vi "I-O Test.vi"() -> ()   [LabVIEW 2019]
uses:
  Classes/Controller/I-O/I-O.lvclass
  Classes/Controller/Controller.lvclass
panel:
  out "channel":dbl
  in  "Type":i32
  in  "Position":i32
  in  "Region":i32
  in  "Value":bool
  in  "Stop":bool
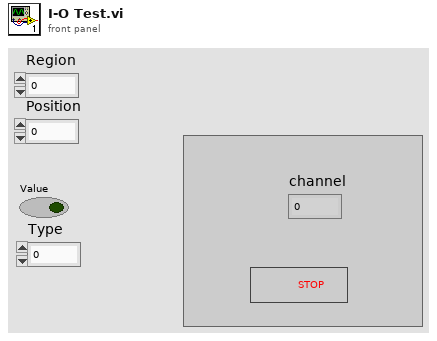
[diagram p1: front panel]
types:
  T1 = typedef "Controller.lvclass/Controllers.ctl" = cluster{"I-O.lvclass":refnum<class "I-O.lvclass">, "Dispenser.lvclass":refnum<class "Dispenser.lvclass">, "Gantry":refnum<k24>}
  T2 = typedef "I-O.lvclass/Pin Map.ctl" = cluster{"Region Valves":i32[], "Extra Valves":dbl[][][], "Tool Primary Valve":i32, "Tool Secondary Valve":i32, "Region Sensors":i32[], "Extra Sensors":dbl[][][], "Tool Primary Sensor":dbl, "Tool Secondary Sensor":dbl, "Compression Sensor":dbl, "5V":i32}
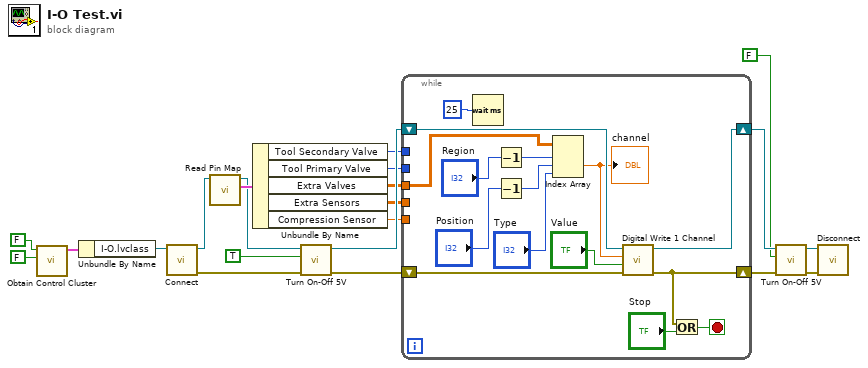
[diagram p0: block diagram]
diagram:
  n1 = call "Obtain Control Cluster.vi"("Dispense"=FALSE, "Motion"=FALSE) -> ("Control Out"=w5:T1)  [unwired: 9 in]
  n2 = Unbundle By Name(w5) -> ("I-O.lvclass"=w4:refnum<class "I-O.lvclass">)
  n3 = call-dynamic "Connect.vi"("Controller in"=w4) -> ("error out"=w12:errorcluster, "Controller out"=w14:refnum<class "I-O.lvclass">)  [unwired: 9 in]
  n4 = call-dynamic "Read Pin Map.vi"("I-O in"=w14) -> ("Pin Map 2"=w16:T2, "I-O out"=w15:refnum<class "I-O.lvclass">)  [unwired: 8 in, 1 out]
  n5 = Unbundle By Name(w16) -> ("Tool Secondary Valve"=w2:i32, "Tool Primary Valve"=w1:i32, "Extra Valves"=w8:dbl[][][], "Extra Sensors"=w13:dbl[][][], "Compression Sensor"=w3:dbl)
  n6 = call-dynamic "Turn On-Off 5V.vi"("error in (no error)"=w12, "Value"=TRUE, "I-O in"=w15) -> ("error out"=w11:errorcluster, "I-O out"=w21:refnum<class "I-O.lvclass">)  [unwired: 7 in]
  n7 = while {
    shift-right: [w31] -> w18
    shift-left: w21 -> [w32]
    tunnel: w13 -> [_]
    shift-right: [w29] -> w10
    shift-left: w11 -> [w30]
    tunnel: w8 -> [w33]
    tunnel: w3 -> [_]
    tunnel: w2 -> [_]
    tunnel: w1 -> [_]
    stop <- w34 stop-if-true
    n8 = Wait (ms)(milliseconds to wait=u32 25) -> ()  [unwired: 1 out]
    n9 = Decrement(x="Region") -> (x-1=w27:i32)
    n10 = Decrement(x="Position") -> (x-1=w24:i32)
    n11 = Index Array(array=w33, index (dim 0)=w27, index (dim 1)=w24, index (dim 2)="Type") -> (element=w22:dbl)
    "channel" <- w22
    n12 = call-dynamic "Digital Write 1 Channel.vi"("error constant"=w30, "Value"="Value", "Channel"=w22, "I-O.lvclass"=w32) -> ("error IO"=w29:errorcluster, "I-O.lvclass 2"=w31:refnum<class "I-O.lvclass">)  [unwired: 6 in]
    n13 = Or(x=w29, y="Stop") -> (x .or. y?=w34:bool)
  }
  n14 = call-dynamic "Turn On-Off 5V.vi"("error in (no error)"=w10, "Value"=FALSE, "I-O in"=w18) -> ("error out"=w9:errorcluster, "I-O out"=w19:refnum<class "I-O.lvclass">)  [unwired: 7 in]
  n15 = call-dynamic "Disconnect.vi"("error in (no error)"=w9, "I-O in"=w19) -> ()  [unwired: 8 in, 1 out]
